vi "Overlay Bodies.vi"(7 "Include Inferred Joints?":bool=TRUE, 8 "error in":errorcluster, 9 "Image":T1, 10 "Body Data":T2[](array[typedef]) {"LeanTrackingState" items=["NotTracked", "Inferred", "Tracked"]; "HandRightState" items=["Unknown", "NotTracked", "Open", "Closed", "Lasso"]; "HandRightConfidence" items=["Low", "High"]; "HandLeftState" items=["Unknown", "NotTracked", "Open", "Closed", "Lasso"]; "HandLeftConfidence" items=["Low", "High"]; "ClippedEdges" items=["None"=0, "Right"=1, "Left"=2, "Top"=4, "Bottom"=8]}) -> (0 "error out":errorcluster, 1 "Image Out":T1)   [LabVIEW 2014]
uses:
  controls/BodyData.ctl
  Microsoft.Kinect
  <vilib>/vision/Image Controls.llb/IMAQ Image.ctl
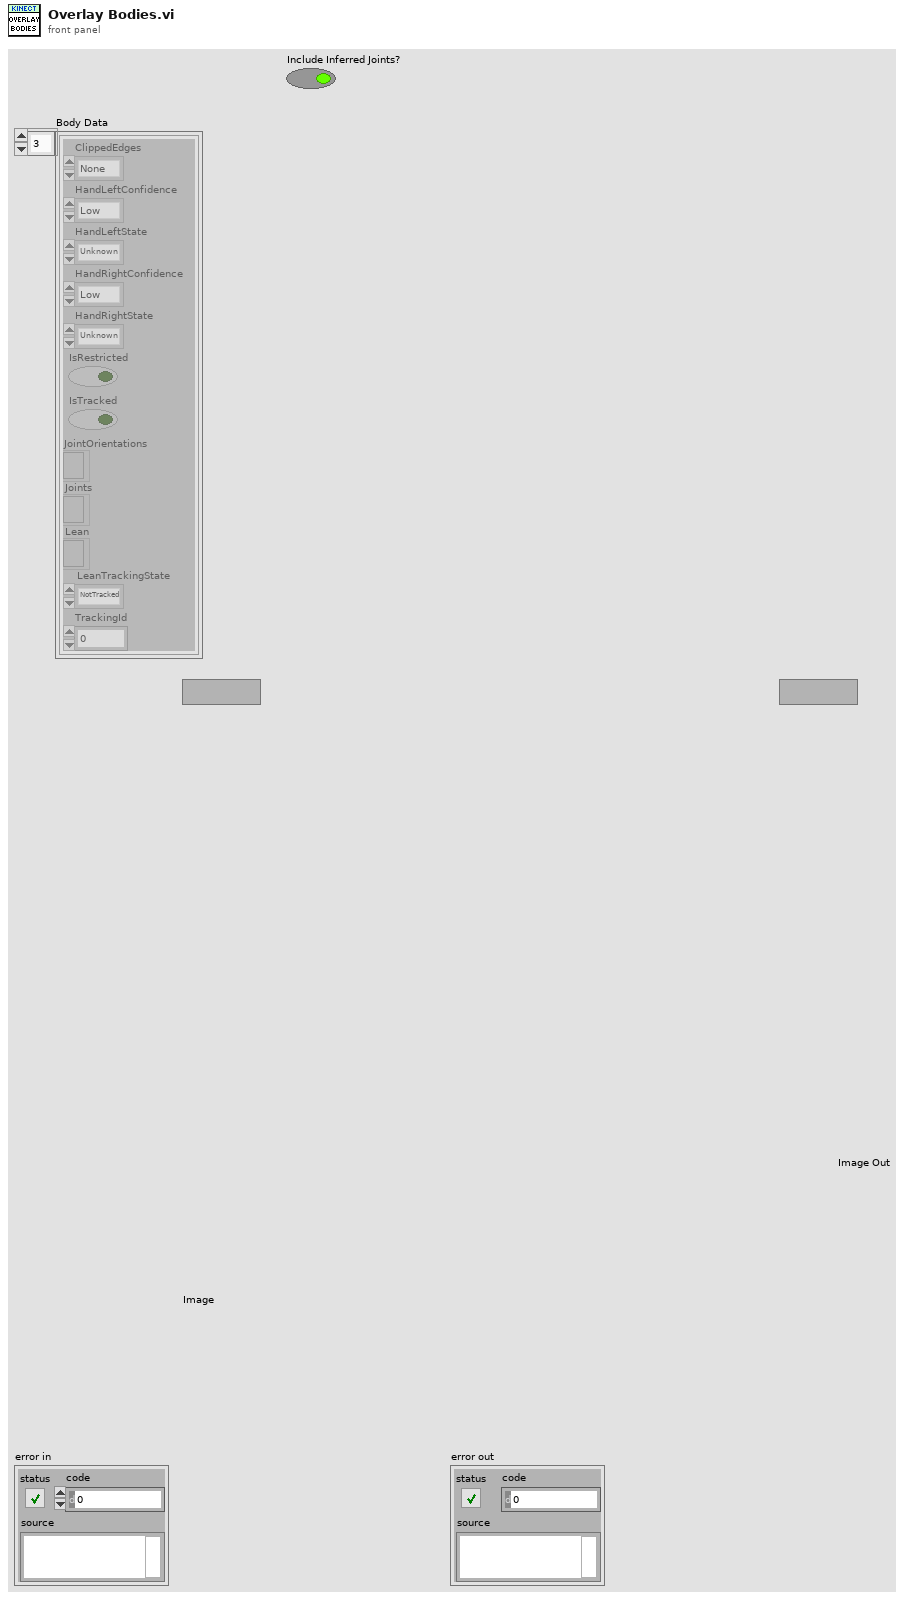
[diagram p1: front panel]
types:
  T1 = typedef "IMAQ Image.ctl" = refnum<image>
  T2 = typedef "BodyData.ctl" = cluster{"ClippedEdges":i32, "HandLeftConfidence":i32, "HandLeftState":i32, "HandRightConfidence":i32, "HandRightState":i32, "IsRestricted":bool, "IsTracked":bool, "JointOrientations":refnum<k24>, "Joints":refnum<k24>, "Lean":refnum<k24>, "LeanTrackingState":i32, "TrackingId":u64}
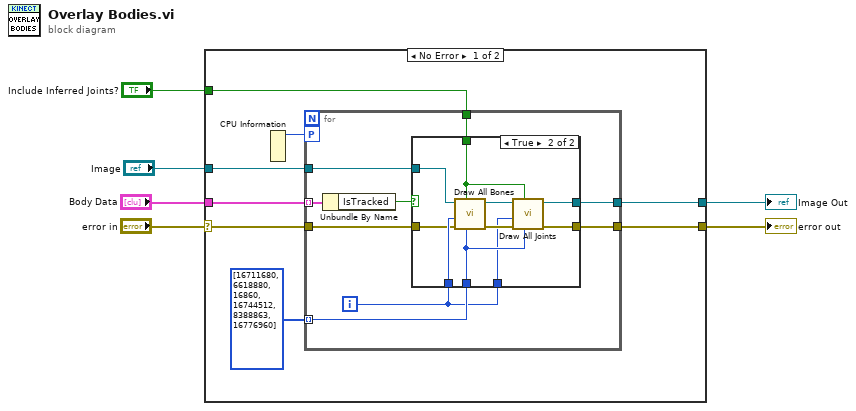
[diagram p0: block diagram]
diagram:
  n1 = case shown="No Error" "error in" {
    selector: "error in" -> [w7 w37]
    tunnel: "Body Data" -> [w14 _]
    tunnel: "Image" -> [w13 w36]
    tunnel: [w12 w37] -> w4
    tunnel: [w11 w36] -> w3
    tunnel: "Include Inferred Joints?" -> [w8 _]
    frame No Error {
      n2 = CPU Information() -> (4:w9:i32)  [unwired: 3 out]
      n3 = for {
        tunnel: w14 -> [w23] mode=indexing
        tunnel: w13 -> [w19]
        tunnel: [w18] -> w11
        tunnel: u32[] [16711680, 6618880, 16860, 16744512, 8388863, 16776960] -> [w17] mode=indexing
        workers-P: w9 -> [_]
        tunnel: w7 -> [w20]
        tunnel: [w21] -> w12
        tunnel: w8 -> [w15]
        i -> [w16]
        n4 = Unbundle By Name(w23) -> ("IsTracked"=w22:bool)
        n5 = case shown="True" w22 {
          tunnel: [w25 w33] -> w21
          tunnel: w20 -> [w25 w26]
          tunnel: w19 -> [w24 w35]
          tunnel: [w24 w31] -> w18
          tunnel: w17 -> [_ w30]
          tunnel: w16 -> [_ w29]
          tunnel: w16 -> [_ w28]
          tunnel: w15 -> [_ w27]
          frame False {
          }
          frame True {
            n6 = call "Draw All Bones.vi"("Color"=w30, "Include Inferred Joints?"=w27, "error in"=w26, "Body Index"=w29, "Image"=w35) -> ("error out"=w34:errorcluster, "Image Out"=w32:T1)  [unwired: 5 in]
            n7 = call "Draw All Joints.vi"("Color"=w30, "Include Inferred Joints?"=w27, "error in (no error)"=w34, "Body Index"=w28, "Image"=w32) -> ("error out"=w33:errorcluster, "Image Out"=w31:T1)  [unwired: 5 in]
          }
        }
      }
    }
    frame Error {
    }
  }
  "error out" <- w4
  "Image Out" <- w3
